vi "InputSN.vi"(9 "上一次测试结果":string, 11 "Sequence Context In":refnum<k7>) -> (0 "error out":errorcluster, 2 "stop":bool=TRUE, 3 "Report Text":string, 10 "Boolean":bool)   [LabVIEW 2018]
panel:
  in  "请输入条码":string
  in  "STOP":bool
  in  "START":bool
  # "请输入/扫描条码"
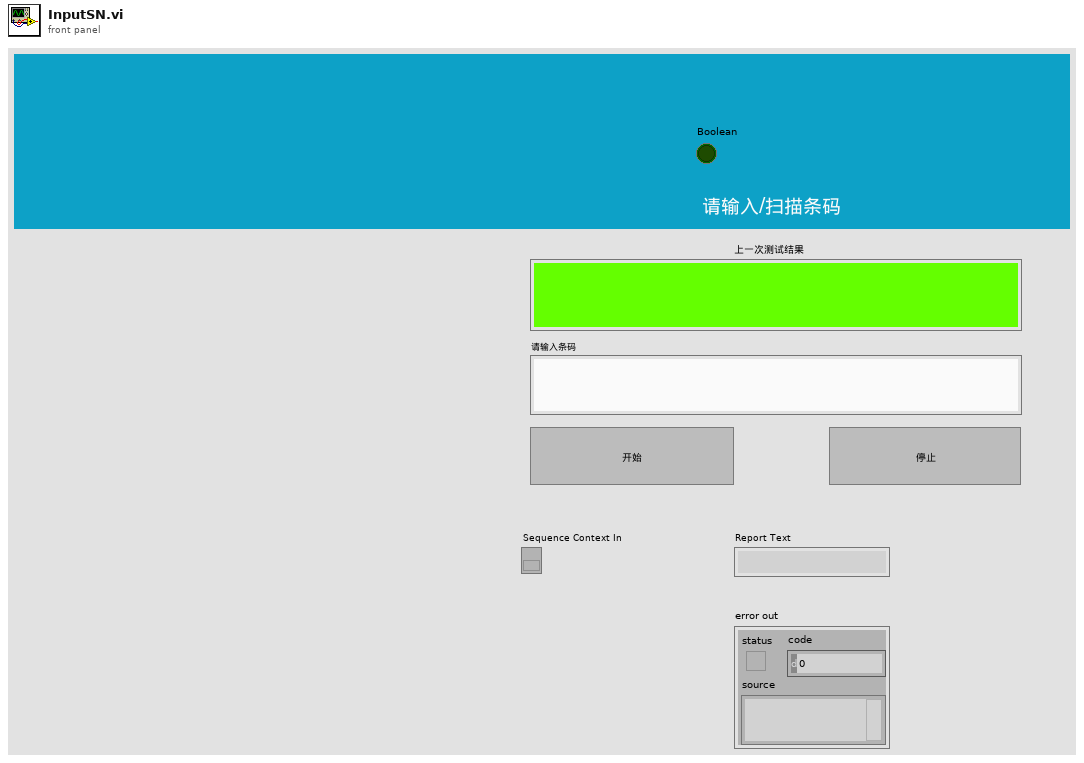
[diagram p1: front panel]
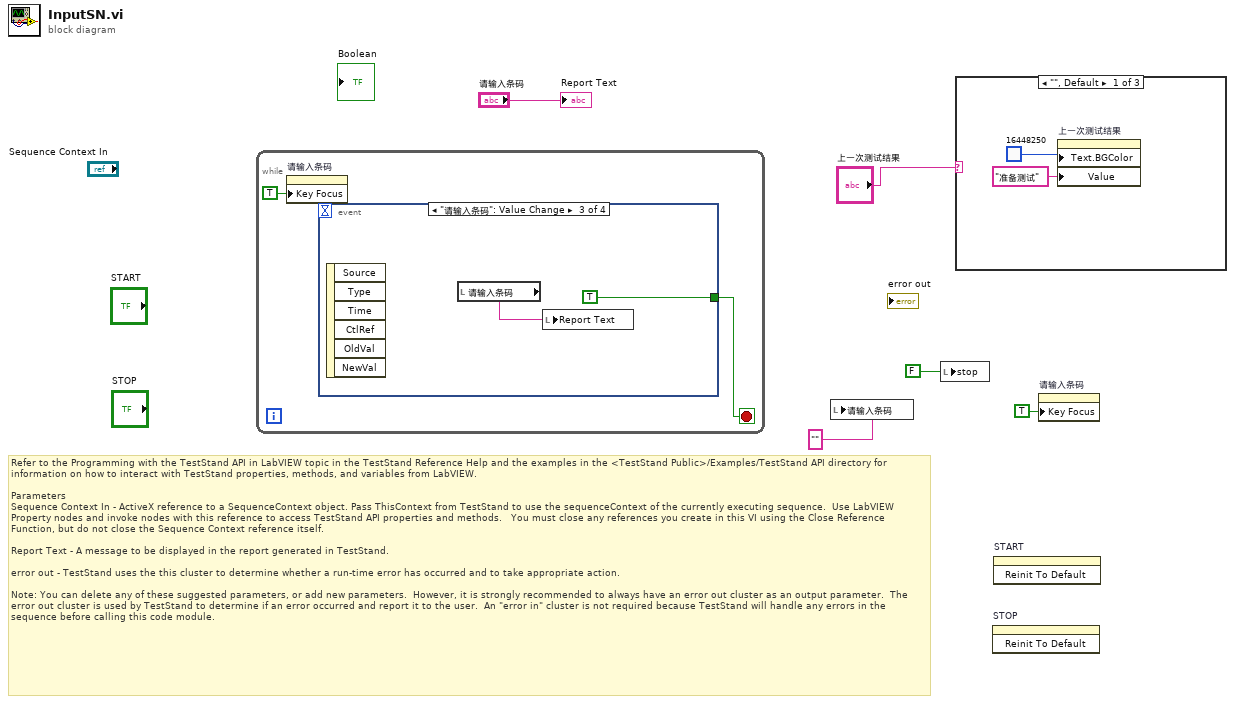
[diagram p0: block diagram]
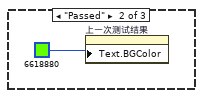
[diagram p2: hidden frame]
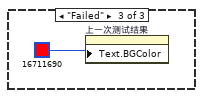
[diagram p3: hidden frame]
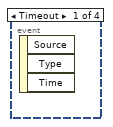
[diagram p4: hidden frame]
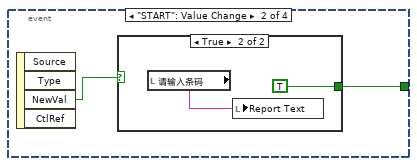
[diagram p5: hidden frame]
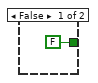
[diagram p6: hidden frame]
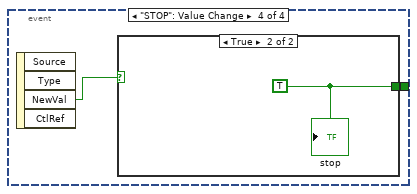
[diagram p7: hidden frame]
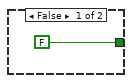
[diagram p8: hidden frame]
diagram:
  # "Refer to the Programming with the TestStand API in LabVIEW topic in the TestStand Reference Help and the examples in the <TestStand Public>/Examples/TestStand API directory for information on how to interact with TestStand properties, methods, and variables from LabVIEW.\n\nParameters\nSequence Context In - ActiveX reference to a SequenceContext object. Pass ThisContext from TestStand to use the sequenceContext of the currently executing sequence.  Use LabVIEW Property nodes and invoke nodes with this reference to access TestStand API properties and methods.   You must close any references you create in this VI using the Close Reference Function, but do not close the Sequence Context reference itself.\n\nReport Text - A message to be displayed in the report generated in TestStand. \n\nerror out - TestStand uses the this cluster to determine whether a run-time error has occurred and to take appropriate action.  \n\nNote: You can delete any of these suggested parameters, or add new parameters.  However, it is strongly recommended to always have an error out cluster as an output parameter.  The error out cluster is used by TestStand to determine if an error occurred and report it to the user.  An \"error in\" cluster is not required because TestStand will handle any errors in the sequence before calling this code module."
  n1 = while {
    stop <- w7 stop-if-true
    n2 = property on="请输入条码" class="Str"("Key Focus"=TRUE) -> ()  [unwired: 2 in, 2 out]
    n3 = event shown="[2] \"请输入条码\": Value Change" {
      selector: _ -> [_ _ _ _]
      dyn-events: _ -> [_ _ _ _]
      timeout: _ -> [_ _ _ _]
      tunnel: [_ w8 TRUE w15] -> w7
      event Timeout {
        n4 = event-data() -> ()  [unwired: 1 in, 3 out]
      }
      event "START": Value Change {
        n5 = event-data() -> ("NewVal"=w9:bool)  [unwired: 1 in, 3 out]
        n6 = case shown="True" w9 {
          tunnel: [FALSE TRUE] -> w8
          frame False {
          }
          frame True {
            n7 = local read "请输入条码"() -> (w11:string)
            n8 = local write "Report Text"(w11) -> ()
          }
        }
      }
      event "请输入条码": Value Change {
        n9 = event-data() -> ()  [unwired: 1 in, 6 out]
        n10 = local read "请输入条码"() -> (w13:string)
        n11 = local write "Report Text"(w13) -> ()
      }
      event "STOP": Value Change {
        n12 = event-data() -> ("NewVal"=w16:bool)  [unwired: 1 in, 3 out]
        n13 = case shown="True" w16 {
          tunnel: [FALSE w18] -> w15
          frame False {
          }
          frame True {
            w18 = TRUE
            "stop" <- w18
          }
        }
      }
    }
  }
  n14 = local write "请输入条码"("" ("请输入条码")) -> ()
  n15 = local write "stop"(FALSE ("Boolean")) -> ()
  n16 = case shown="\"\", Default" "上一次测试结果" {
    frame "", Default {
      n17 = property on="上一次测试结果" class="Str"("Text.BGColor"=u32 16448250, "Value"="准备测试" ("上一次测试结果")) -> ()  [unwired: 2 in, 2 out]
    }
    frame "Passed" {
      n18 = property on="上一次测试结果" class="Str"("Text.BGColor"=u32 6618880) -> ()  [unwired: 2 in, 2 out]
    }
    frame "Failed" {
      n19 = property on="上一次测试结果" class="Str"("Text.BGColor"=u32 16711690) -> ()  [unwired: 2 in, 2 out]
    }
  }
  n20 = invoke on="STOP" class="Bool (strict)" method="Reinit To Default"() -> ()  [unwired: 3 in, 3 out]
  n21 = invoke on="START" class="Bool (strict)" method="Reinit To Default"() -> ()  [unwired: 3 in, 3 out]
  n22 = property on="请输入条码" class="Str"("Key Focus"=TRUE) -> ()  [unwired: 2 in, 2 out]
  "Report Text" <- "请输入条码"
